vi "LS DAS Global.vi"(0 "Recording In":bool, 1 "Bank2Slow In":bool, 2 "Mode":T2(ring), 5 "Initial LS Data In":T1={"Total Cycles"=[0, 0, 0, 0, 0, 0, 0, 0, 0, 0, 0, 0], "Steps"=[0, 0, 0, 0, 0, 0, 0, 0, 0, 0, 0, 0], "Anomalies Total"=[0, 0, 0, 0, 0, 0, 0, 0, 0, 0, 0, 0], "Cycles"=[0, 0, 0, 0, 0, 0, 0, 0, 0, 0, 0, 0], "Anomalies/Cycle"=[0, 0, 0, 0, 0, 0, 0, 0, 0, 0, 0, 0], "Anomalies (Last Cycle)"=[0, 0, 0, 0, 0, 0, 0, 0, 0, 0, 0, 0], "Opens"=[0, 0, 0, 0, 0, 0, 0, 0, 0, 0, 0, 0]} {"Opens" format="%#.0f"; "Anomalies (Last Cycle)" format="%#.0f"; "Anomalies/Cycle" format="%#.0f"; "Cycles" format="%#.0f"; "Anomalies Total" format="%#.0f"; "Steps" format="%#.0f"; "Total Cycles" format="%#.0f"}, 7 "LS Cluster In":T3, 9 "SDfree":i64, 11 "SDmax'":i64, 12 "Note IN":string) -> (3 "Bank2Slow Out":bool, 4 "Recording Out":bool, 6 "Initial LS Data Out":T1 {"Opens" format="%#.0f"; "Anomalies (Last Cycle)" format="%#.0f"; "Anomalies/Cycle" format="%#.0f"; "Cycles" format="%#.0f"; "Anomalies Total" format="%#.0f"; "Steps" format="%#.0f"; "Total Cycles" format="%#.0f"}, 8 "LS Cluster Out":T3, 10 "SD%":dbl, 14 "Note Out":string, 15 "Note Active":bool)   [LabVIEW 2018]
uses:
  Type Defs/LS Data.ctl
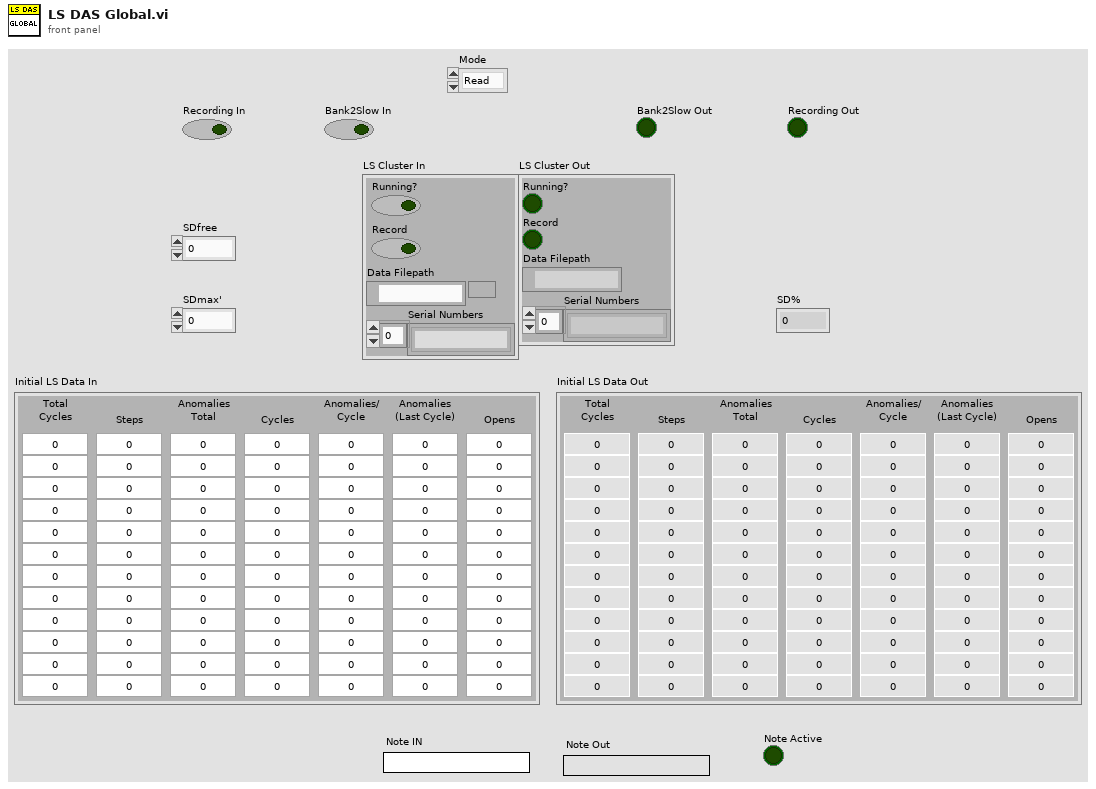
[diagram p1: front panel]
types:
  T1 = typedef "LS Data.ctl" = cluster{"Total Cycles":u32[], "Steps":u32[], "Anomalies Total":i32[], "Cycles":u32[], "Anomalies/Cycle":i32[], "Anomalies (Last Cycle)":i32[], "Opens":i32[]}
  T2 = enum16{"Read", "Engine Writes", "Main Writes", "Write Anomalies", "Write Init Data", "Write Storage", "Write Note", "Read Note"}
  T3 = cluster{"Running?":bool, "Record":bool, "Data Filepath":path, "Serial Numbers":string[]}
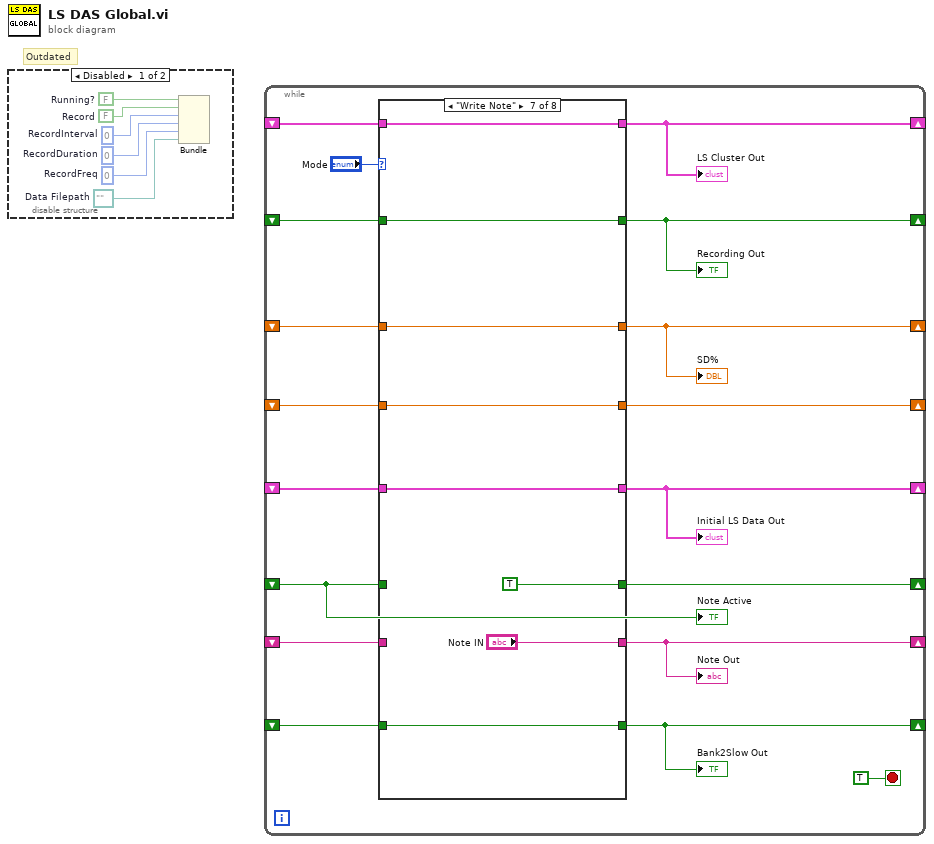
[diagram p0: block diagram]
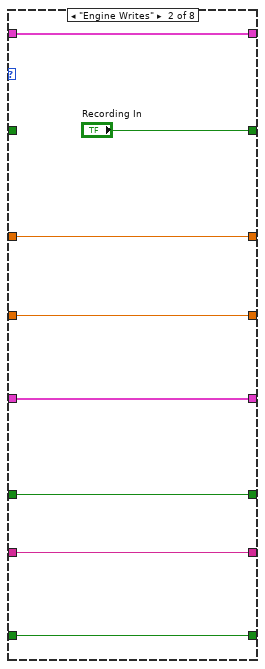
[diagram p4: hidden frame]
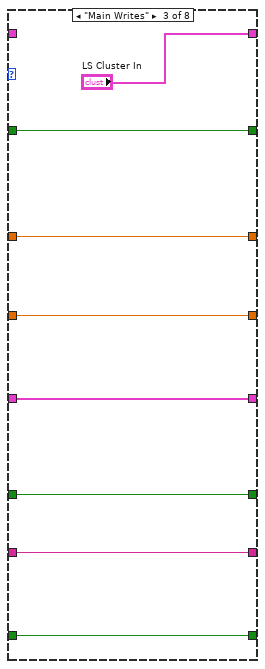
[diagram p5: hidden frame]
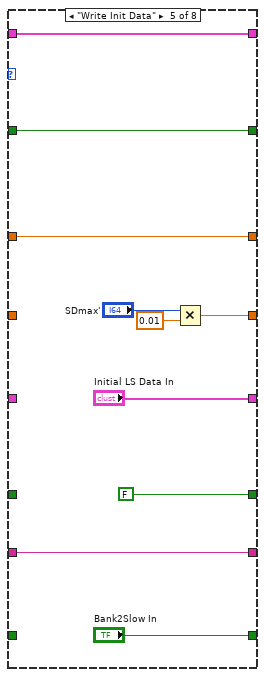
[diagram p7: hidden frame]
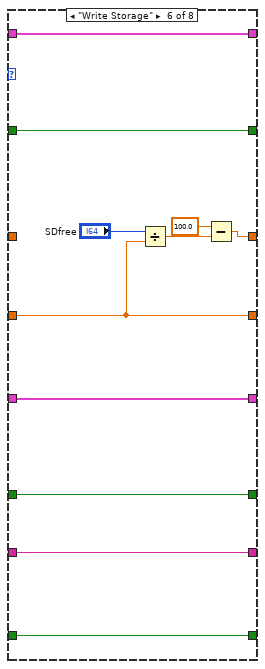
[diagram p8: hidden frame]
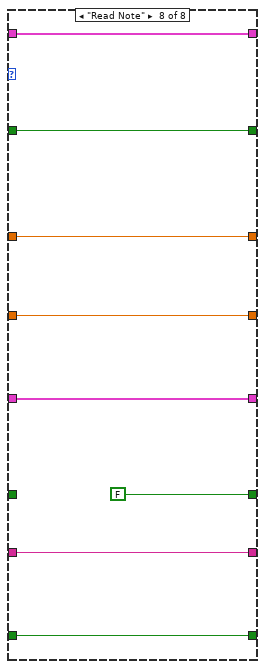
[diagram p9: hidden frame]
diagram:
  # "Outdated"
  n1 = disable-structure shown="Disabled" {
    frame Disabled {
      w1 = path ""  # Data Filepath
      w2 = 0  # RecordFreq
      w3 = 0  # RecordDuration
      w4 = 0  # RecordInterval
      w5 = FALSE  # Record
      w6 = FALSE  # Running?
      n2 = Bundle("Running?"=w6, "Record"=w5, "RecordInterval"=w4, "RecordDuration"=w3, "RecordFreq"=w2, "Data Filepath"=w1) -> ()  [unwired: 1 in, 1 out]
    }
    frame Enabled {
    }
  }
  n3 = while {
    shift-right: [w22] -> _
    shift-left: _ -> [w23]
    shift-right: [w19] -> _
    shift-left: _ -> [w20]
    shift-right: [w17] -> _
    shift-left: _ -> [w18]
    shift-right: [w16] -> _
    shift-left: _ -> [w15]
    shift-right: [w14] -> _
    shift-left: _ -> [w13]
    shift-right: [w10] -> _
    shift-left: _ -> [w11]
    shift-right: [w12] -> _
    shift-left: _ -> [w9]
    shift-right: [w7] -> _
    shift-left: _ -> [w8]
    stop <- TRUE stop-if-true
    n4 = case shown="\"Write Note\"" "Mode" {
      tunnel: w23 -> [w32 w40 _ w55 w64 w77 w85 w93]
      tunnel: [w32 w40 "LS Cluster In" w55 w64 w77 w85 w93] -> w22
      tunnel: w20 -> [w31 _ w47 w56 w65 w76 w84 w92]
      tunnel: [w31 "Recording In" w47 w56 w65 w76 w84 w92] -> w19
      tunnel: [w30 w38 w46 w54 "Initial LS Data In" w75 w81 w89] -> w17
      tunnel: w18 -> [w30 w38 w46 w54 _ w75 w81 w89]
      tunnel: [w29 w37 w45 w53 w61 w73 w82 w90] -> w16
      tunnel: w15 -> [w29 w37 w45 w53 _ w73 w82 w90]
      tunnel: [w28 w36 w44 w52 w60 w70 w83 w91] -> w14
      tunnel: w13 -> [w28 w36 w44 w52 w60 _ w83 w91]
      tunnel: [w27 w35 w43 w51 FALSE w69 TRUE FALSE] -> w12
      tunnel: [w26 w34 w42 w50 w58 w68 "Note IN" w88] -> w10
      tunnel: w11 -> [w26 w34 w42 w50 w58 w68 _ w88]
      tunnel: w9 -> [w27 w35 w43 w51 _ w69 _ _]
      tunnel: [w25 w33 w41 w49 "Bank2Slow In" w67 w78 w86] -> w7
      tunnel: w8 -> [w25 w33 w41 w49 _ w67 w78 w86]
      frame "Read", Default {
      }
      frame "Engine Writes" {
      }
      frame "Main Writes" {
      }
      frame "Write Anomalies" {
      }
      frame "Write Init Data" {
        n5 = Multiply(x="SDmax'", y=0.01) -> (x*y=w61:dbl)
      }
      frame "Write Storage" {
        n6 = Divide(x="SDfree", y=w73) -> (x/y=w71:dbl)
        n7 = Subtract(x=100.0, y=w71) -> (x-y=w70:dbl)
      }
      frame "Write Note" {
      }
      frame "Read Note" {
      }
    }
    "LS Cluster Out" <- w22
    "Recording Out" <- w19
    "Initial LS Data Out" <- w17
    "SD%" <- w14
    "Note Out" <- w10
    "Bank2Slow Out" <- w7
    "Note Active" <- w9
  }
